vi "Generate Mapping Error Name.vi"(8 "error in":errorcluster, 11 "Type":T1) -> (0 "error out":errorcluster, 3 "String":string)   [LabVIEW 2020, in "Modbus Master System Explorer.lvlib"]
uses:
  Modbus Master System Explorer.lvlib
  Modbus Type.ctl
  Shared/Modbus Master Shared.lvlib
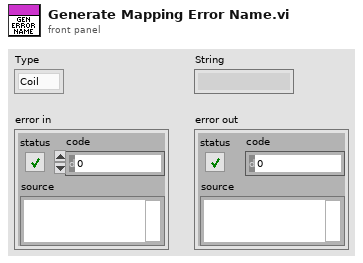
[diagram p1: front panel]
types:
  T1 = typedef "Modbus Master Shared.lvlib/Modbus Type.ctl" = enum16{"Coil", "Discrete Input", "Holding Register", "Input Register"}
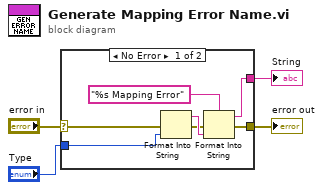
[diagram p0: block diagram]
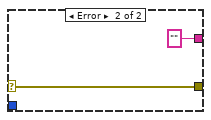
[diagram p2: hidden frame]
diagram:
  n1 = case shown="No Error" "error in" {
    selector: "error in" -> [w10 w13]
    tunnel: [w11 ""] -> w4
    tunnel: "Type" -> [w7 _]
    tunnel: [w5 w13] -> w1
    frame No Error {
      n2 = Format Into String(error in=w10, w7) -> (resulting string=w9:string, error out=w6:errorcluster)  [unwired: 2 in]
      n3 = Format Into String(format string="%s Mapping Error", error in=w6, w9) -> (resulting string=w11:string, error out=w5:errorcluster)  [unwired: 1 in]
    }
    frame Error {
    }
  }
  "String" <- w4
  "error out" <- w1
